vi "Sparge_subVI_BM.vi"(8 "BitNum":u32=4, 9 "BoardNum":u32, 11 "Sparge now":bool=TRUE) -> (3 "Sparging":bool)   [LabVIEW 2021]
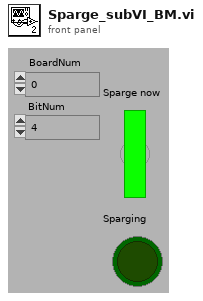
[diagram p1: front panel]
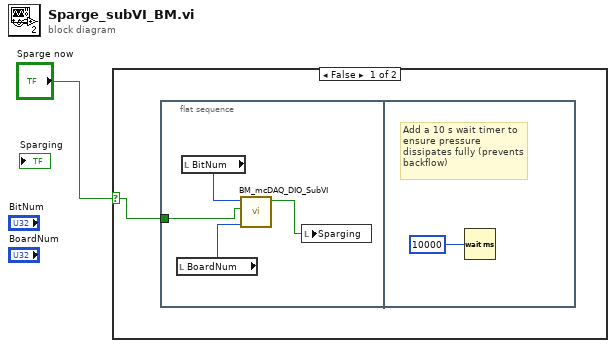
[diagram p0: block diagram]
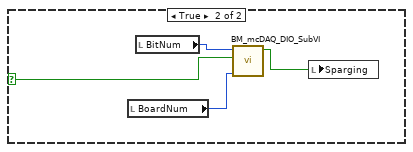
[diagram p2: hidden frame]
diagram:
  n1 = case shown="False" "Sparge now" {
    selector: "Sparge now" -> [w2 w10]
    frame False {
      n2 = flat-sequence {
        tunnel: w2 -> [w5]
        frame #0 {
          n3 = local read "BoardNum"() -> (w3:u32)
          n4 = local read "BitNum"() -> (w4:u32)
          n5 = call "BM_mcDAQ_DIO_SubVI.vi"("BoardNum"=w3, "BitValue"=w5, "BitNum"=w4) -> ("Control out"=w6:bool)  [unwired: 8 in]
          n6 = local write "Sparging"(w6) -> ()
        }
        frame #1 {
          # "Add a 10 s wait timer to ensure pressure dissipates fully (prevents backflow)"
          n7 = Wait (ms)(milliseconds to wait=u32 10000) -> ()  [unwired: 1 out]
        }
      }
    }
    frame True {
      n8 = local read "BoardNum"() -> (w8:u32)
      n9 = local read "BitNum"() -> (w9:u32)
      n10 = call "BM_mcDAQ_DIO_SubVI.vi"("BoardNum"=w8, "BitValue"=w10, "BitNum"=w9) -> ("Control out"=w11:bool)  [unwired: 8 in]
      n11 = local write "Sparging"(w11) -> ()
    }
  }
